vi "Dresser DXD Build Command String.vi"(3 "Input Value (\"\")":string, 4 "Command Mnemonic (\"\")":string, 5 "DXD Address (1)":T1=1 min=1 max=99 step=1) -> (2 "Command String":string)   [LabVIEW 2015]
doc: "This VI builds the command string to be sent to the Dresser DXD Series pressure transducer. Inputs are DXD Address, Command Mnemonic, Input Value (for write only). The required '#' start character preceeds the command and a carriage return termination character is appended to the end.\n\nThe command string returned is in the following format:\n\nStart DXD Command Input Value Termination\nCharacter Address Mnumonic (for write only) Character\n-----------------------------------------------------------------------------------------------------------------------------------\n# 01 - 99 2 Character Alpha Alphanumeric CR\n\n\nWritten by:\nBLOOMY CONTROLS, INC\nWINDSOR, CT 06095, USA\n860-298-9925\nwww.bloomy.com\nV2.0.0\nMay, 2002"
uses:
  Type Defs/DXD Address.ctl
panel:
  # "For instructions on the use of this VI, press Ctrl+H to display the help window and move the mouse over the icon, controls, and indicators"
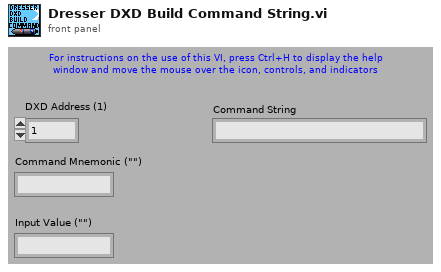
[diagram p1: front panel]
types:
  T1 = typedef "DXD Address.ctl" = i32
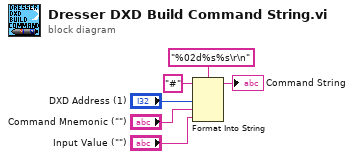
[diagram p0: block diagram]
diagram:
  n1 = Format Into String(format string="%02d%s%s\r\n" ("Format String"), initial string="#" ("Input String"), "DXD Address (1)", "Command Mnemonic (\"\")", "Input Value (\"\")") -> (resulting string=→"Command String":string)  [unwired: 1 in, 1 out]
